vi "Edit Data.vi"(2 "error in (no error)":errorcluster, 3 "History Data input":T2) -> (0 "error out":errorcluster, 1 "History Data output":T2)   [LabVIEW 2021]
doc: "Este VI se encarga de editar/recortar los datos de temperatura"
panel:
  in  "Quit":bool
  in  "Edit button":bool
  in  "Posicion final":dbl
  in  "Posicion inicial":dbl
  out "Temperature Data":T1(graph)
  # "Elige con que tramo quedarte y toma pasos múltiplos de 0,5"
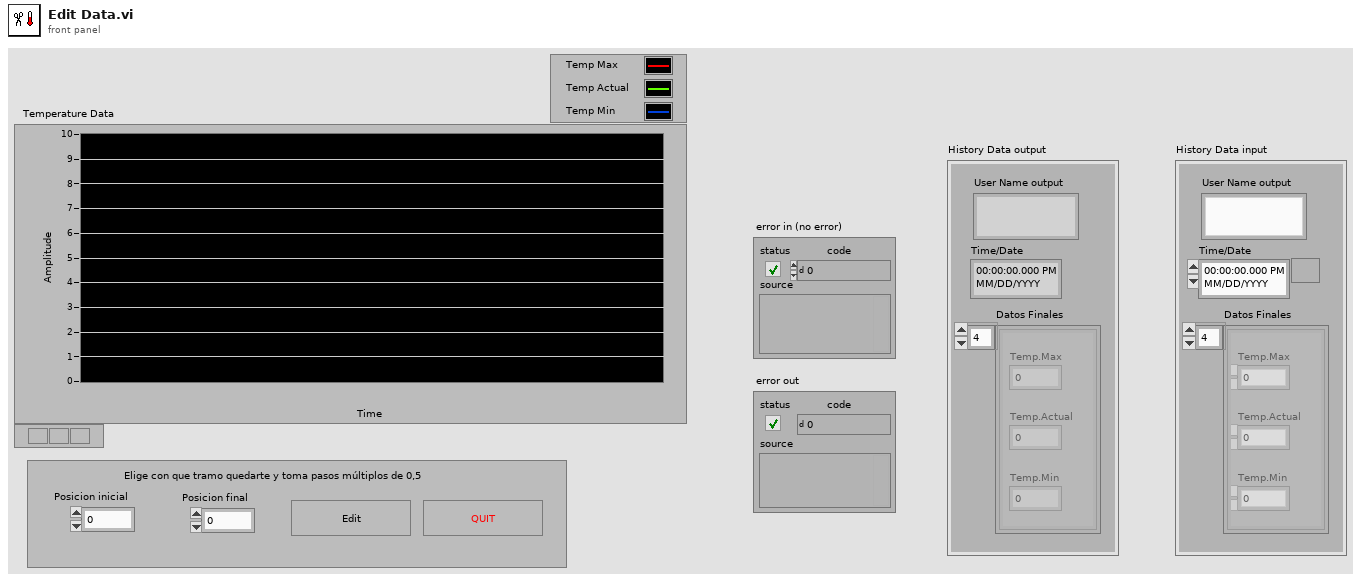
[diagram p1: front panel]
types:
  T1 = cluster{"Temp.Max":dbl, "Temp.Actual":dbl, "Temp.Min":dbl}[]
  T2 = cluster{"User Name output":string, "Time/Date":timestamp, "Datos Finales":cluster{"Temp.Max":dbl, "Temp.Actual":dbl, "Temp.Min":dbl}[]}
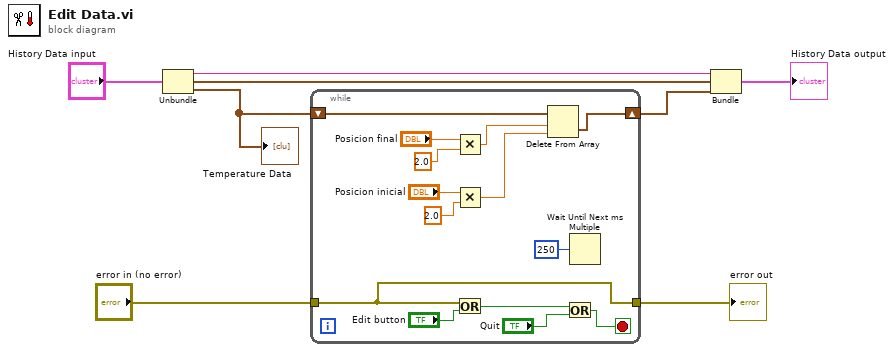
[diagram p0: block diagram]
diagram:
  n1 = Unbundle("History Data input") -> ("User Name output"=w7:string, "Time/Date"=w6:timestamp, "Datos Finales"=w1:T1)
  "Temperature Data" <- w1
  n2 = while {
    tunnel: [w15] -> w5
    tunnel: "error in (no error)" -> [w15]
    shift-right: [w10] -> w3
    shift-left: w1 -> [w9]
    stop <- w11 stop-if-true
    n3 = Multiply(x="Posicion final", y=2.0) -> (x*y=w21:dbl)
    n4 = Multiply(x="Posicion inicial", y=2.0) -> (x*y=w19:dbl)
    n5 = Or(x=w15, y="Edit button") -> (x .or. y?=w13:bool)
    n6 = Delete From Array(array=w9, length=w21, index=w19) -> (deleted portion=w10:T1)  [unwired: 1 out]
    n7 = Or(x=w13, y="Quit") -> (x .or. y?=w11:bool)
    n8 = Wait Until Next ms Multiple(millisecond multiple=u32 250 ("millisecond timer value")) -> ()  [unwired: 1 out]
  }
  "error out" <- w5
  n9 = Bundle("User Name output"=w7, "Time/Date"=w6, "Datos Finales"=w3) -> (→"History Data output":T2)  [unwired: 1 in]
